vi "list.get_video.vi"(8 "error in (no error)":errorcluster, 10 "index":i32, 11 "List in":refnum<class "List.lvclass">) -> (0 "error out":errorcluster, 2 "Video":refnum<class "Video.lvclass">, 3 "List out":refnum<class "List.lvclass">)   [LabVIEW 2020, in "List.lvclass"]
uses:
  List.lvclass
  Asset/Asset.lvclass/Asset.ctl
  List.lvclass/List.ctl
  Video/Video.lvclass
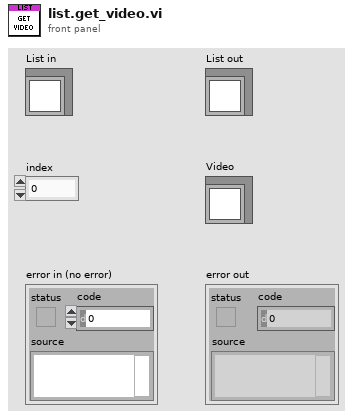
[diagram p1: front panel]
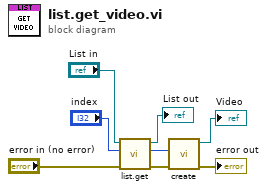
[diagram p0: block diagram]
diagram:
  n1 = call "list.get.vi"("error in"="error in (no error)", "index"="index", "List in"="List in") -> ("error out"=w3:errorcluster, "handle"=w4:i32, "List out"=→"List out":refnum<class "List.lvclass">)  [unwired: 6 in]
  n2 = call "create.vi"("error in (no error)"=w3, "handle"=w4) -> ("error out"=→"error out":errorcluster, "Video"=→"Video":refnum<class "Video.lvclass">)  [unwired: 8 in]
